vi "Read IV Settings.vi"(8 "error in (no error)":errorcluster, 11 "Dot Settings in":refnum<class "Dot Settings.lvclass">) -> (0 "error out":errorcluster, 2 "IV Settings":T1, 3 "Dot Settings out":refnum<class "Dot Settings.lvclass">)   [LabVIEW 2019, in "Dot Settings.lvclass"]
uses:
  Dot Settings.lvclass
  TypeDefs/IV Settings.ctl
  Dot Settings.lvclass/Dot Settings.ctl
  5b696732-5c78-441d-b330-2aec1c2f6ac1.vi
  <vilib>/JDP Science/JSONtext/JSON text to Variant.vi
  <vilib>/JDP Science/JSONtext/LVClass Serializer/JSONtext LVClass Serializer.lvclass
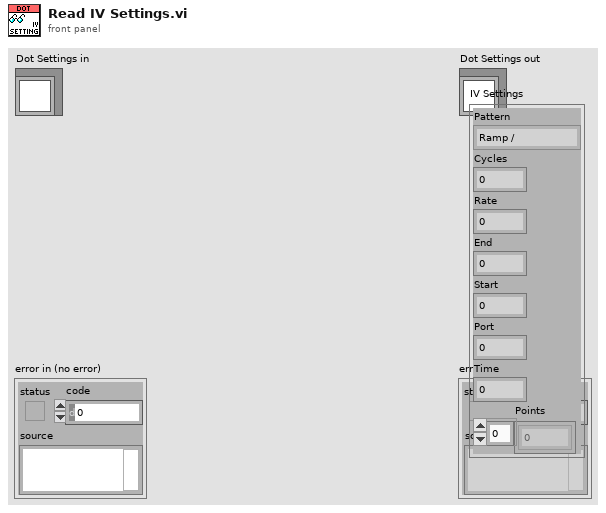
[diagram p1: front panel]
types:
  T1 = typedef "Dot Settings.lvclass/IV Settings.ctl" = cluster{"Pattern":enum16{"Ramp /", "Ramp /\\", "Smooth Ramp _/", "Smooth Ramp _/\\_", "Frequency"}, "Cycles":i32, "Rate":dbl, "End":dbl, "Start":dbl, "Port":u32, "Time":dbl, "Points":dbl[]}
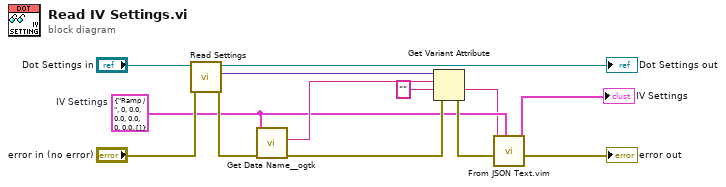
[diagram p0: block diagram]
diagram:
  w3 = T1 {"Pattern"=enum."Ramp /", "Cycles"=0, "Rate"=0.0, "End"=0.0, "Start"=0.0, "Port"=0, "Time"=0.0, "Points"=[]}  # IV Settings
  n1 = call "Read Settings.vi"("error in (no error)"="error in (no error)", "Dot Settings in"="Dot Settings in") -> ("error out"=w7:errorcluster, "Settings"=w11:variant, "Dot Settings out"=→"Dot Settings out":refnum<class "Dot Settings.lvclass">)  [unwired: 7 in]
  n2 = call <userlib>:"Get Data Name__ogtk.vi"("error in (no error)"=w7, "Data"=w3) -> ("error out"=w9:errorcluster, "Data Name"=w10:string)  [unwired: 7 in, 1 out]
  n3 = Get Variant Attribute(Variant=w11, name=w10, default value (empty Variant)="", error in=w9) -> (value=w1:string, error out=w5:errorcluster)  [unwired: 2 out]
  n4 = call "From JSON Text.vim"("Data Type and Default Value"=w3, "error in (no error)"=w5, "JSON"=w1) -> ("error out"=→"error out":errorcluster, "Data out"=→"IV Settings":T1)  [unwired: 7 in]
